vi "Get Strings From Enum.vi"(8 "错误输入":errorcluster, 10 "Enum":variant) -> (0 "错误输出":errorcluster, 1 "String Value":string, 2 "Enum Strings":string[](array[string]), 3 "Enum Name":string)   [LabVIEW 2012, in "TD Tools.lvlib"]
uses:
  TD Tools.lvlib
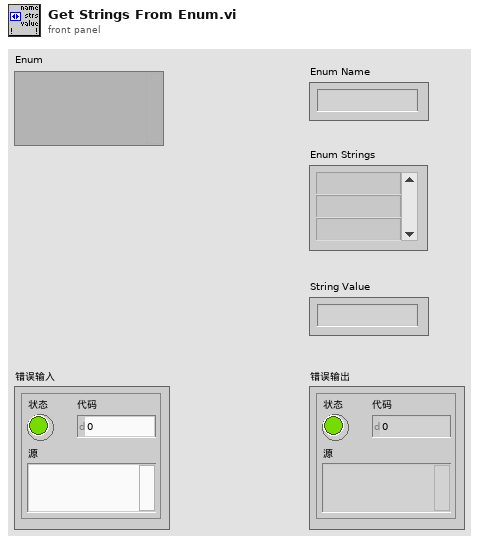
[diagram p1: front panel]
types:
  T1 = typedef "TD Tools.lvlib/Type Descriptor.ctl" = u16[]
  T2 = typedef "TD Tools.lvlib/Type Descriptor Header.ctl" = cluster{"length":u16, "private":u8, "type":T3, "# elements":u16}
  T3 = typedef "TD Tools.lvlib/Type Descriptor Enumeration.ctl" = enum16{"<Null>", "I8", "I16", "I32", "I64", "U8", "U16", "U32", "U64", "SGL", "DBL", "EXT", "CSG", "CDB", "CXT", "0x0F", "0x10", "0x11", "0x12", "0x13", "0x14", "Enum U8", "Enum U16", "Enum U32", "Enum U64", "SGL PQ", "DBL PQ", "EXT PQ", "CSG PQ", "CDB PQ", "CXT PQ", "0x1F", "0x20", "Boolean", "0x22", "0x23", "0x24", "0x25", "0x26", "0x27", "0x28", "0x29", "0x2A", "0x2B", "0x2C", "0x2D", "0x2E", "0x2F", "String", "0x31", "Path", "Pict", "0x34", "0x35", "0x36", "DAQ", "0x38", "0x39", "0x3A", "0x3B", "0x3C", "0x3D", "0x3E", "0x3F", "Array", "0x41", "0x42", "0x43", "0x44", "0x45", "0x46", "0x47", "0x48", "0x49", "0x4A", "0x4B", "0x4C", "0x4D", "0x4E", "0x4F", "Cluster", "0x51", "0x52", "Variant", "Waveform", "0x55", "0x56", "0x57", "0x58", "0x59", "0x5A", "0x5B", "0x5C", "0x5D", "0x5E", "0x5F", "0x60", "0x61", "0x62", "0x63", "0x64", "0x65", "0x66", "0x67", "0x68", "0x69", "0x6A", "0x6B", "0x6C", "0x6D", "0x6E", "0x6F", "Refnum"}
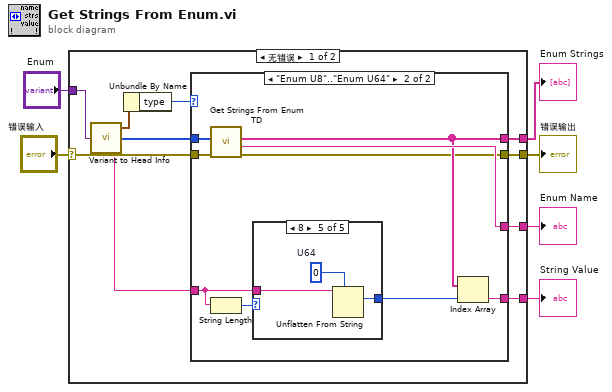
[diagram p0: block diagram]
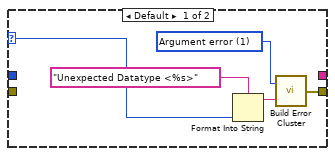
[diagram p2: hidden frame]
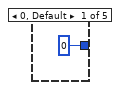
[diagram p3: hidden frame]
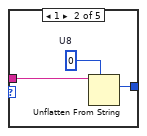
[diagram p4: hidden frame]
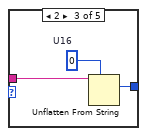
[diagram p5: hidden frame]
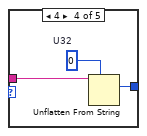
[diagram p6: hidden frame]
diagram:
  n1 = case shown="无错误" "错误输入" {
    selector: "错误输入" -> [w11 w44]
    tunnel: "Enum" -> [w16 _]
    tunnel: [w13 w44] -> w4
    tunnel: [w10 _] -> w3
    tunnel: [w9 _] -> w2
    tunnel: [w7 _] -> w1
    frame No Error {
      n2 = call "Variant to Head Info.vi"("Variant"=w16) -> ("Data String"=w8:string, "Type Descriptor"=w12:T1, "Type Descriptor Header"=w15:T2)  [unwired: 2 in]
      n3 = Unbundle By Name(w15) -> ("type"=w14:T3)
      n4 = case shown="\"Enum U8\"..\"Enum U64\"" w14 {
        selector: w14 -> [w18 _]
        tunnel: [w17 w22] -> w13
        tunnel: w12 -> [_ w30]
        tunnel: w11 -> [_ w29]
        tunnel: [_ w28] -> w10
        tunnel: [_ w24] -> w9
        tunnel: w8 -> [_ w26]
        tunnel: [_ w23] -> w7
        frame Default {
          w19 = 1 items=["No error", "Argument error", "Memory is full", "Out of zone", "End of file", "File already open", "Generic file I/O error", "File not found", "File permission error", "Disk is full", "Duplicate path", "Too many files open", "System feature not enabled", "Resource file not found", "Cannot add resource", "Resource not found", "Image not found", "Image memory error", "Pen does not exist", "Config type invalid", "Config token not found", "Config parse error", "Config memory error", "Bad external code format", "Bad external code offset", "External code not present", "Null window", "Destroy window error", "Null menu", "Print aborted", "Bad print record", "Print driver error", "Windows error during printing", "Memory error during printing", "Print dialog error", "Generic print error", "Invalid device refnum", "Device not found", "Device parameter error", "Device unit error", "Cannot open device", "Device call aborted", "Generic error", "Cancelled by user", "Object ID too low", "Object ID too high", "Object not in heap", "Unknown heap", "Unknown object (invalid DefProc)", "Unknown object (DefProc not in table)", "Message out of range", "Invalid (null) method", "Unknown message", "Manager call not supported", "Bad address", "Network operation in progress", "Network operation timed out", "Connection is busy", "Network attribute not supported", "Network error", "Address in use", "System out of memory", "Connection aborted", "Connection refused", "Not connected", "Already connected", "Connection closed", "Initialization error (interapplication manager)", "Bad occurrence", "Wait on unbound occurrence handler", "Occurrence queue overflow", "Datalog type conflict", "Unused", "Unrecognized type (interapplication manager)", "Memory corrupt", "Failed to make temporary DLL", "Old CIN version", "Drag socket not found", "Failed to load drop-object", "Failed to register OLE object", "Failed to release OLE object", "Format specifier type mismatch", "Unknown format specifier", "Too few format specifiers", "Too many format specifiers", "Scan failed", "Newer CIN version", "Error converting to variant", "Runtime menu error", "Password tampered", "Variant attribute not found", "Incompatible variant data type", "Event data is not available", "Event Store is not present", "Occurrence is not found", "Event Queue is not created", "Event info is not available", "Refnum passed is NULL", "Error retrieving Class GUID", "Error retrieving CoClass GUID", "Error retrieving TypeLib GUID.", "Bad built application magic bytes.", "Specific driver is different from the specific driver associated with the Logical Name.", "There is no session opened to the class driver.", "Max Error", "MAX - Error with config objects", "MAX - Error loading configuration", "MAX - Group not supported"]
          n5 = Format Into String(format string="Unexpected Datatype <%s>" ("Format String"), w18) -> (resulting string=w21:string)  [unwired: 2 in, 1 out]
          n6 = call "Build Error Cluster.vi"("String to Prepend to source (\"\")"=w21, "code"=w19) -> ("error out"=w17:errorcluster)
        }
        frame "Enum U8".."Enum U64" {
          n7 = call "Get Strings From Enum TD.vi"("错误输入"=w29, "Type Descriptor"=w30) -> ("错误输出"=w22:errorcluster, "Enum Name"=w28:string, "Enum Strings"=w24:string[])  [unwired: 7 in]
          n8 = String Length(string=w26) -> (length=w27:i32)
          n9 = case shown="8" w27 {
            tunnel: w26 -> [_ w34 w37 w40 w41]
            tunnel: [u32 0 ("U32") w32 w35 w38 w42] -> w25
            frame 0, Default {
            }
            frame 1 {
              w33 = u8 0  # U8
              n10 = Unflatten From String(type=w33, binary string=w34) -> (value=w32:u8)  [unwired: 3 in, 2 out]
            }
            frame 2 {
              w36 = u16 0  # U16
              n11 = Unflatten From String(type=w36, binary string=w37) -> (value=w35:u16)  [unwired: 3 in, 2 out]
            }
            frame 4 {
              w39 = u32 0  # U32
              n12 = Unflatten From String(type=w39, binary string=w40) -> (value=w38:u32)  [unwired: 3 in, 2 out]
            }
            frame 8 {
              w43 = u64 0  # U64
              n13 = Unflatten From String(type=w43, binary string=w41) -> (value=w42:u64)  [unwired: 3 in, 2 out]
            }
          }
          n14 = Index Array(array=w24, index=w25) -> (element=w23:string)
        }
      }
    }
    frame Error {
    }
  }
  "Enum Name" <- w3
  "Enum Strings" <- w2
  "String Value" <- w1
  "错误输出" <- w4
